vi "decrementMonth.vi"(8 "error in (no error)":errorcluster, 11 "WhichMonth in":refnum<class "WhichMonth.lvclass">) -> (0 "error out":errorcluster, 3 "WhichMonth out":refnum<class "WhichMonth.lvclass">)   [LabVIEW 2018, in "WhichMonth.lvclass"]
uses:
  WhichMonth.lvclass
  WhichMonth.lvclass/WhichMonth.ctl
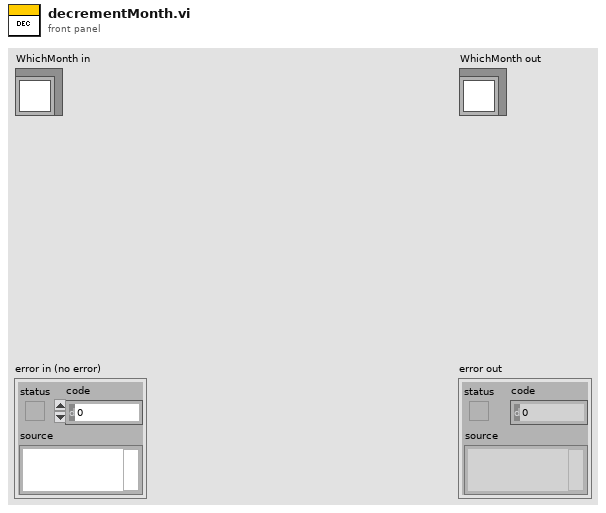
[diagram p1: front panel]
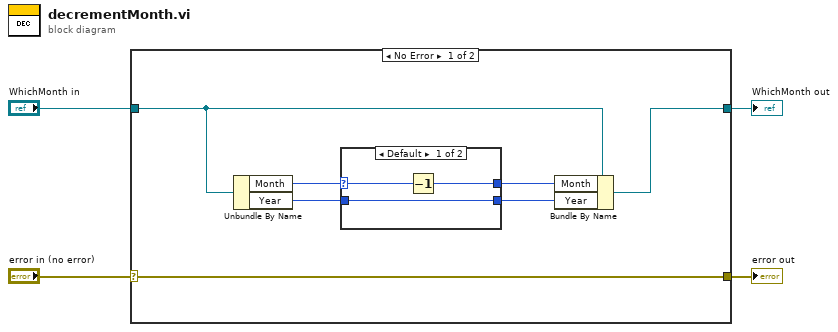
[diagram p0: block diagram]
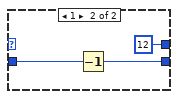
[diagram p2: hidden frame]
diagram:
  n1 = case shown="No Error" "error in (no error)" {
    selector: "error in (no error)" -> [w11 w19]
    tunnel: [w11 w19] -> w3
    tunnel: [w7 w18] -> w1
    tunnel: "WhichMonth in" -> [w8 w18]
    frame No Error {
      n2 = Unbundle By Name(w8) -> ("Month"=w10:i32, "Year"=w9:i32)
      n3 = case shown="Default" w10 {
        selector: w10 -> [w14 _]
        tunnel: w9 -> [w13 w17]
        tunnel: [w13 w16] -> w5
        tunnel: [w12 12] -> w6
        frame Default {
          n4 = Decrement(x=w14) -> (x-1=w12:i32)
        }
        frame 1 {
          n5 = Decrement(x=w17) -> (x-1=w16:i32)
        }
      }
      n6 = Bundle By Name(cluster=w8, "Month"=w6, "Year"=w5) -> (w7:refnum<class "WhichMonth.lvclass">)
    }
    frame Error {
    }
  }
  "error out" <- w3
  "WhichMonth out" <- w1
